vi "Fit Multi-Gaus Peaks.vi"(4 "Function":enum16{"Gauss", "Lorentz"}(ring), 5 "Window end":dbl=697.0, 6 "Repeat":i32, 7 "Window start":dbl=690.0, 9 "Guess":T1(array[cluster]), 10 "Y":dbl[](array[numeric]), 11 "X":dbl[](array[numeric])) -> (1 "Fit":T1(array[cluster]), 2 "Fit plot":cluster{"Array":dbl[], "Array":dbl[]})   [LabVIEW 2016]
uses:
  <vilib>/Analysis/NI_AALPro.lvlib
  Smooth Background DBL.vi
panel:
  in  "Use last fit as  guess":bool
  out "errors":i32[](array[numeric])
  in  "Filter background":bool
  out "Result":T2
  out "error":i32
  out "XY Graph":cluster{"all rows":dbl[], "Data out":dbl[]}[](graph)
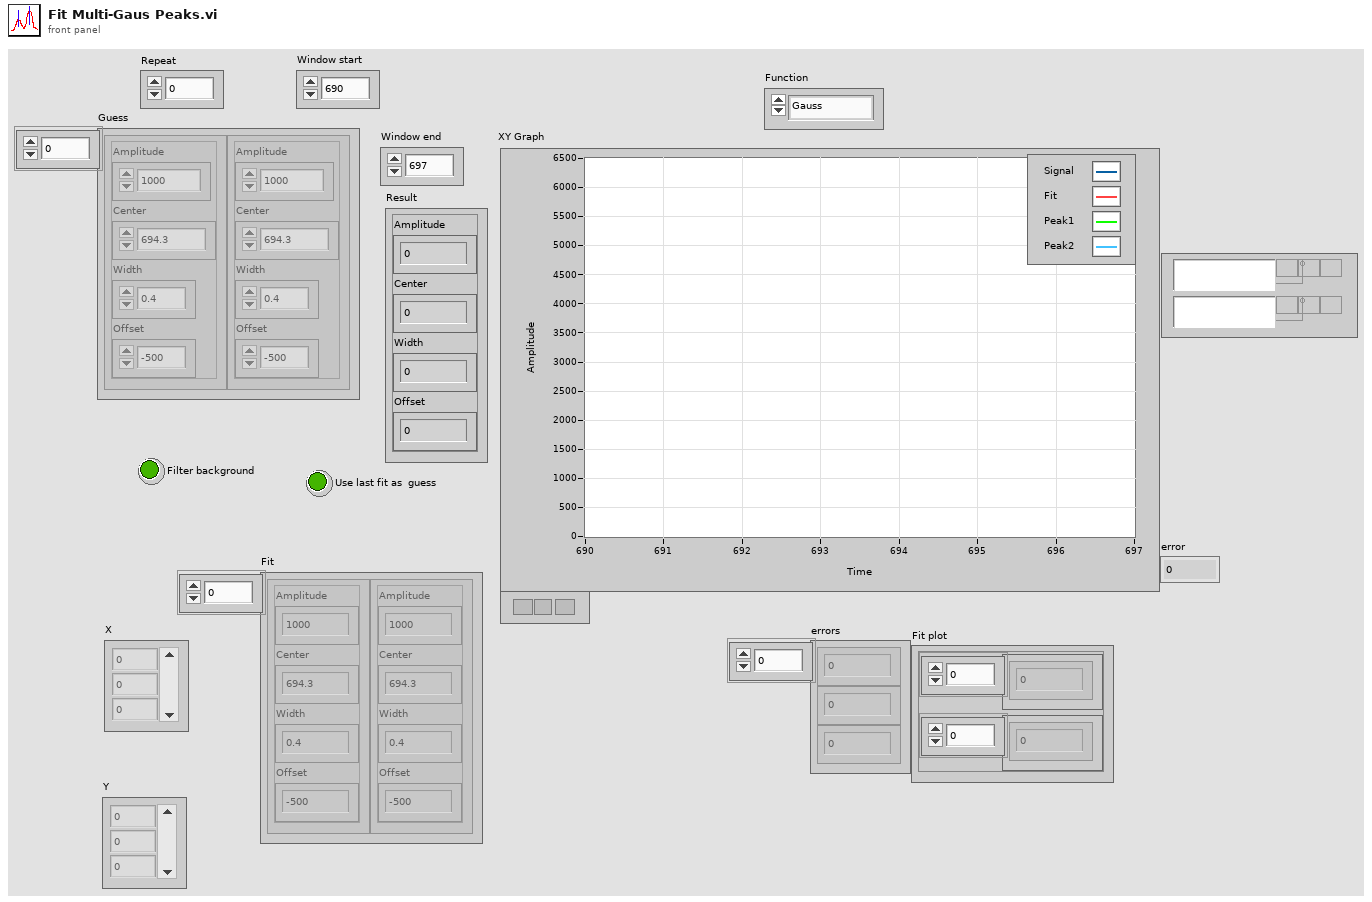
[diagram p1: front panel]
types:
  T1 = cluster{"Amplitude":dbl, "Center":dbl, "Width":dbl, "Offset":dbl}[]
  T2 = cluster{"Amplitude":dbl, "Center":dbl, "Width":dbl, "Offset":dbl}
  T3 = cluster{"amp min":dbl, "amp max":dbl, "center min":dbl, "center max":dbl, "deviation min":dbl, "deviation max":dbl, "offset min":dbl, "offset max":dbl}
  T4 = enum16{"Lowpass", "Highpass", "Bandpass", "Bandstop"}
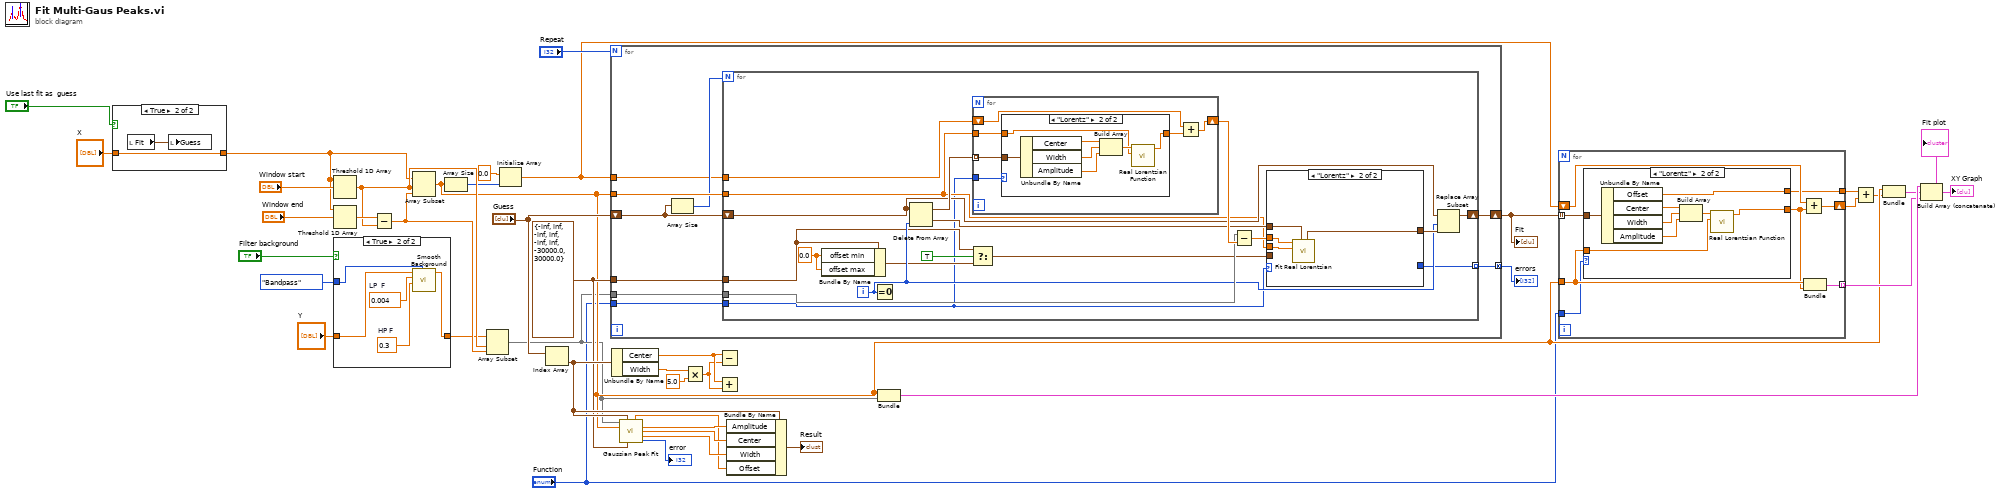
[diagram p0: block diagram]
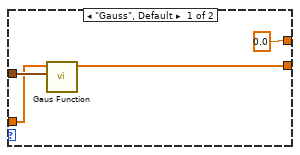
[diagram p3: hidden frame]
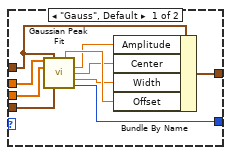
[diagram p4: hidden frame]
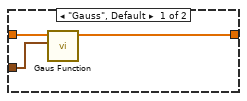
[diagram p5: hidden frame]
diagram:
  w16 = T3 {"amp min"=-inf, "amp max"=inf, "center min"=-inf, "center max"=inf, "deviation min"=-inf, "deviation max"=inf, "offset min"=-30000.0, "offset max"=30000.0} ("parameter bounds")
  n1 = case shown="True" "Use last fit as  guess" {
    tunnel: "X" -> [w42 w43]
    tunnel: [w42 w43] -> w3
    frame False {
    }
    frame True {
      n2 = local read "Fit"() -> (w44:T1)
      n3 = local write "Guess"(w44) -> ()
    }
  }
  n4 = Threshold 1D Array(2:"Window start", 3:w3) -> (0:w36:dbl)  [unwired: 1 in]
  n5 = Threshold 1D Array(2:"Window end", 3:w3) -> (0:w37:dbl)  [unwired: 1 in]
  n6 = case shown="True" "Filter background" {
    tunnel: T4."Bandpass" ("Type") -> [_ w50]
    tunnel: "Y" -> [w45 w47]
    tunnel: [w45 w46] -> w34
    frame False {
    }
    frame True {
      w48 = 0.3  # HP F
      w49 = 0.004  # LP  F
      n7 = call-poly "Smooth Background.vi"("Type"=w50, "HP F"=w48, "LP  F"=w49, "Data"=w47) -> ("Data out"=w46:dbl[])  [unwired: 6 in, 1 out]
    }
  }
  n8 = Subtract(x=w37, y=w36) -> (x-y=w35:dbl)
  n9 = Array Subset(array=w3, index=w36, length=w35) -> (w11:dbl[])
  n10 = Array Size(array=w11) -> (size(s)=w19:i32)
  n11 = Array Subset(array=w34, index=w36, length=w35) -> (w9:dbl[])
  n12 = Initialize Array(0.0 ("element"), w19) -> (w13:dbl[])
  n13 = Index Array(array="Guess") -> (element=w21:T2)  [unwired: 1 in]
  n14 = for {
    N: "Repeat" -> [_]
    shift-right: [w54] -> w15
    shift-left: "Guess" -> [w58]
    tunnel: w11 -> [w59]
    tunnel: w13 -> [w56]
    tunnel: w9 -> [w55]
    tunnel: w16 -> [w53]
    tunnel: [w52] -> w8 mode=concatenating
    tunnel: "Function" -> [w51]
    n15 = Array Size(array=w58) -> (size(s)=w57:i32)
    n16 = for {
      N: w57 -> [_]
      tunnel: w59 -> [w61]
      tunnel: w56 -> [w76]
      tunnel: w55 -> [w74]
      shift-right: [w69] -> w54
      shift-left: w58 -> [w72]
      tunnel: w53 -> [w67]
      tunnel: [w63] -> w52 mode=indexing
      tunnel: w51 -> [w60]
      i -> [w68]
      w64 = 0.0
      n17 = Bundle By Name(cluster=w67, "offset min"=w64, "offset max"=w64) -> (w66:T3)
      n18 = Equal To 0?(x=w68) -> ()  [unwired: 1 out]
      n19 = Delete From Array(array=w72, index=w68) -> (deleted portion=w71:T2, array with subset deleted=w77:T1)  [unwired: 1 in]
      n20 = Select(t=w67, s=TRUE, f=w66) -> (s? t:f=w65:T3)
      n21 = for {
        tunnel: w77 -> [w97] mode=indexing
        tunnel: w61 -> [w96]
        shift-right: [w93] -> w75
        shift-left: w76 -> [w95]
        tunnel: w60 -> [w92]
        n22 = case shown="\"Lorentz\"" w92 {
          tunnel: w97 -> [w100 w104]
          tunnel: w96 -> [w99 w101]
          tunnel: [w98 w103] -> w94
          frame "Gauss", Default {
            n23 = call "Gaus Function.vi"("Fit params"=w100, "X"=w99) -> ("Y"=w98:dbl[])  [unwired: 9 in]
          }
          frame "Lorentz" {
            n24 = Unbundle By Name(w104) -> ("Center"=w107:dbl, "Width"=w106:dbl, "Amplitude"=w105:dbl)
            n25 = Build Array(w107, w106, w105) -> (w102:dbl[])
            n26 = call "Real Lorentzian Function.vi"("X"=w101, "a"=w102) -> ("f(X,a)"=w103:dbl[])  [unwired: 2 in, 2 out]
          }
        }
        n27 = Add(x=w95, y=w94) -> (x+y=w93:dbl[])
      }
      n28 = Subtract(x=w74, y=w75) -> (x-y=w73:dbl[])
      n29 = case shown="\"Lorentz\"" w60 {
        tunnel: w73 -> [w87 w91]
        tunnel: w71 -> [w86 w89]
        tunnel: [w81 w88] -> w70
        tunnel: w65 -> [w80 _]
        tunnel: [w79 _] -> w63
        tunnel: w61 -> [w78 w90]
        frame "Gauss", Default {
          n30 = call <vilib>:"Gaussian Peak Fit.vi"("Y"=w87, "initial guess"=w86, "X"=w78, "parameter bounds"=w80) -> ("offset"=w85:dbl, "amplitude"=w84:dbl, "center"=w83:dbl, "standard deviation"=w82:dbl, "error"=w79:i32)  [unwired: 5 in, 2 out]
          n31 = Bundle By Name(cluster=w86, "Amplitude"=w84, "Center"=w83, "Width"=w82, "Offset"=w85) -> (w81:T2)
        }
        frame "Lorentz" {
          n32 = call "Fit Real Lorentzian.vi"("Initial guess"=w89, "X"=w90, "Y"=w91) -> ("Fit"=w88:T2)  [unwired: 8 in]
        }
      }
      n33 = Replace Array Subset(array=w72, new element=w70, index=w68) -> (w69:T1)
    }
  }
  "Fit" <- w15
  "errors" <- w8
  n34 = Unbundle By Name(w21) -> ("Center"=w32:dbl, "Width"=w33:dbl)
  n35 = call <vilib>:"Gaussian Peak Fit.vi"("Y"=w9, "initial guess"=w21, "X"=w11, "parameter bounds"=w16) -> ("offset"=w26:dbl, "amplitude"=w29:dbl, "center"=w28:dbl, "standard deviation"=w27:dbl, "error"=→"error":i32)  [unwired: 5 in, 2 out]
  n36 = Multiply(x=w33, y=5.0) -> (x*y=w30:dbl)
  n37 = Subtract(x=w32, y=w30) -> ()  [unwired: 1 out]
  n38 = Add(x=w32, y=w30) -> ()  [unwired: 1 out]
  n39 = Bundle By Name(cluster=w21, "Amplitude"=w29, "Center"=w28, "Width"=w27, "Offset"=w26) -> (→"Result":T2)
  n40 = Bundle(w11, w9) -> (w39:cluster{dbl[], dbl[]})  [unwired: 1 in]
  n41 = for {
    tunnel: [w115] -> w14 mode=indexing
    tunnel: w11 -> [w112]
    tunnel: w15 -> [w110] mode=indexing
    shift-right: [w113] -> w12
    shift-left: w13 -> [w114]
    tunnel: "Function" -> [w109]
    tunnel: [w108] -> w1
    n42 = case shown="\"Lorentz\"" w109 {
      tunnel: w110 -> [w119 w124]
      tunnel: w112 -> [w118 w123]
      tunnel: [w117 w121] -> w111
      tunnel: [0.0 ("Offset") w120] -> w108
      frame "Gauss", Default {
        n43 = call "Gaus Function.vi"("Fit params"=w119, "X"=w118) -> ("Y"=w117:dbl[])  [unwired: 9 in]
      }
      frame "Lorentz" {
        n44 = Unbundle By Name(w124) -> ("Offset"=w120:dbl, "Center"=w127:dbl, "Width"=w126:dbl, "Amplitude"=w125:dbl)
        n45 = Build Array(w127, w126, w125) -> (w122:dbl[])
        n46 = call "Real Lorentzian Function.vi"("X"=w123, "a"=w122) -> ("f(X,a)"=w121:dbl[])  [unwired: 2 in, 2 out]
      }
    }
    n47 = Add(x=w114, y=w111) -> (x+y=w113:dbl[])
    n48 = Bundle(w112, "f(X,a)"=w111) -> (w115:cluster{dbl[], "f(X,a)":dbl[]})  [unwired: 1 in]
  }
  n49 = Add(x=w1, y=w12) -> (x+y=w2:dbl[])
  n50 = Bundle(w11, w2) -> (w10:cluster{dbl[], dbl[]})  [unwired: 1 in]
  "Fit plot" <- w10
  n51 = Build Array (concatenate)(w39, w10, w14) -> (→"XY Graph":cluster{dbl[], "f(X,a)":dbl[]}[])
